vi "experiment description to file name Samuel.vi"(11 "Experiment Description":T1={"GAL4 Line / Line A / Genotype"="CS", "UAS-Effector Line / Line B"="", "Experiment Type"=enum."olfaction", "Stimulus Descriptions"=[{"Stimulus Modulation"=enum."Spatial", "stimulant"="co2", "maximum"=5, "mimimum"=0, "period"=20, "Modulation Detail"=enum."LinearX", "unit"="pct", "period_unit"="cm", "additional description"=enum."none", "description"=""}], "other name"="", "Training/Habituation Pre Exposure"={"CS"="", "UCS"="", "Training Protocol"="", "Training ID Code"="", "Training Type"=enum."none (no directory)"}}) -> (1 "data directory with time":path, 2 "filename":string, 3 "data directory":path)   [LabVIEW 2013]
panel:
  out "error out":errorcluster
  in  "error in":errorcluster
  # "X"
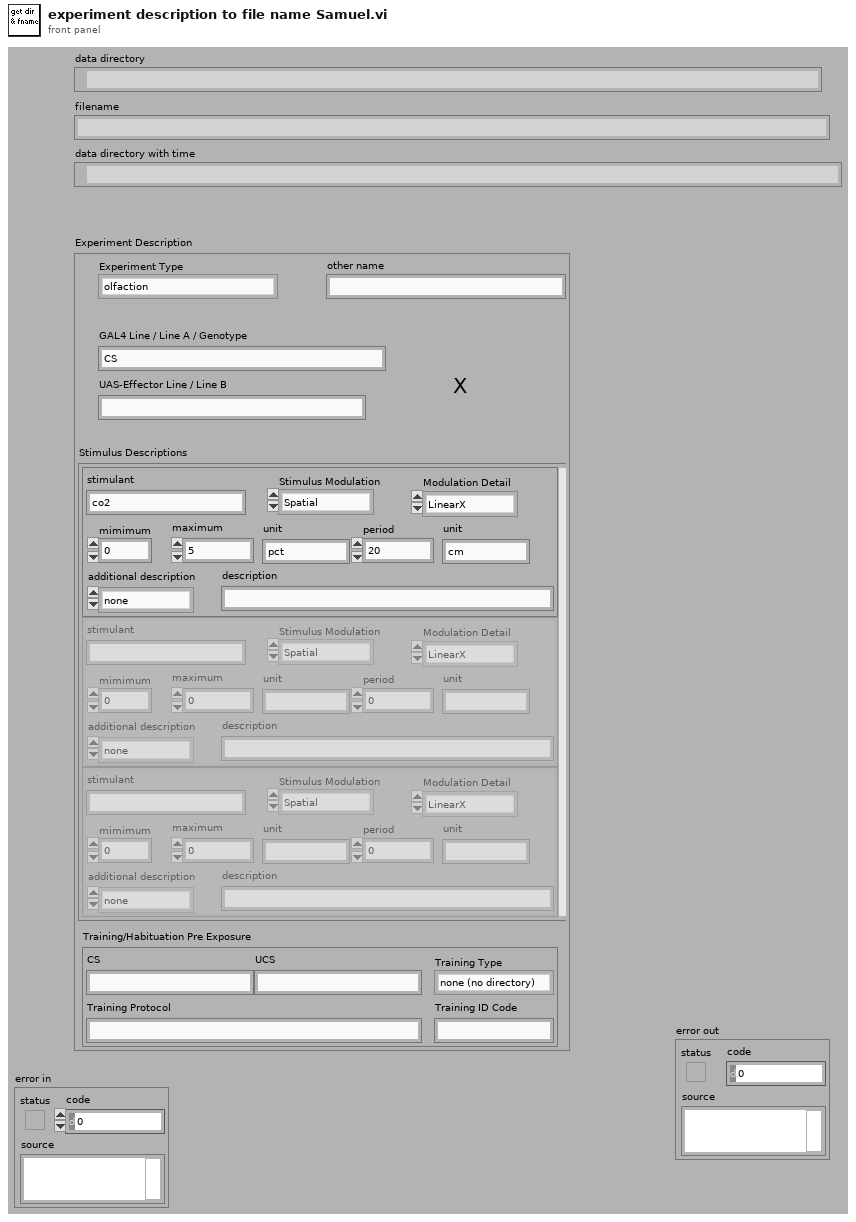
[diagram p1: front panel]
types:
  T1 = cluster{"GAL4 Line / Line A / Genotype":string, "UAS-Effector Line / Line B":string, "Experiment Type":enum16{"other", "olfaction", "phototaxis", "chemotaxis", "thermotaxis", "multi sensory"}, "Stimulus Descriptions":cluster{"Stimulus Modulation":enum16{"Spatial", "Temporal", "Constant", "Other"}, "stimulant":string, "maximum":u16, "mimimum":u16, "period":u16, "Modulation Detail":enum16{"LinearX", "LinearY", "Triangle", "Sine", "Square", "AngledX", "AngledY"}, "unit":string, "period_unit":string, "additional description":enum16{"none", "append", "replace"}, "description":string}[], "other name":string, "Training/Habituation Pre Exposure":cluster{"CS":string, "UCS":string, "Training Protocol":string, "Training ID Code":string, "Training Type":enum16{"none (no directory)", "untrained", "trained"}}}
  T2 = enum16{"other", "olfaction", "phototaxis", "chemotaxis", "thermotaxis", "multi sensory"}
  T3 = cluster{"Stimulus Modulation":enum16{"Spatial", "Temporal", "Constant", "Other"}, "stimulant":string, "maximum":u16, "mimimum":u16, "period":u16, "Modulation Detail":enum16{"LinearX", "LinearY", "Triangle", "Sine", "Square", "AngledX", "AngledY"}, "unit":string, "period_unit":string, "additional description":enum16{"none", "append", "replace"}, "description":string}[]
  T4 = cluster{"CS":string, "UCS":string, "Training Protocol":string, "Training ID Code":string, "Training Type":enum16{"none (no directory)", "untrained", "trained"}}
  T5 = enum16{"none (no directory)", "untrained", "trained"}
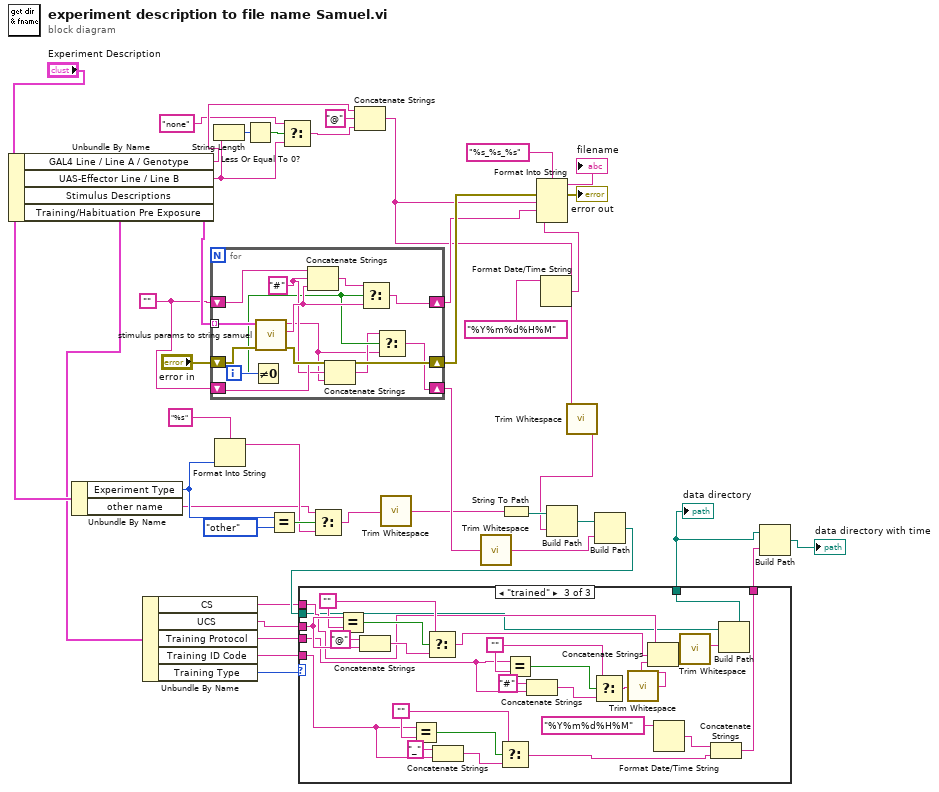
[diagram p0: block diagram]
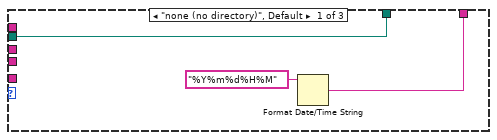
[diagram p2: hidden frame]
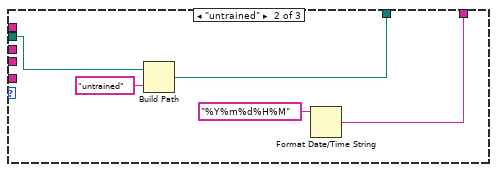
[diagram p3: hidden frame]
diagram:
  w20 = "" ("stimulus string description")
  n1 = Unbundle By Name("Experiment Description") -> ("GAL4 Line / Line A / Genotype"=w9:string, "UAS-Effector Line / Line B"=w4:string, "Stimulus Descriptions"=w41:T3, "Training/Habituation Pre Exposure"=w19:T4)
  n2 = Unbundle By Name("Experiment Description") -> ("Experiment Type"=w26:T2, "other name"=w21:string)
  n3 = Unbundle By Name(w19) -> ("CS"=w13:string, "UCS"=w12:string, "Training Protocol"=w11:string, "Training ID Code"=w10:string, "Training Type"=w18:T5)
  n4 = for {
    tunnel: w41 -> [w56] mode=indexing
    shift-right: [w54] -> w31
    shift-left: w20 -> [w53]
    shift-right: [w51] -> w39
    shift-left: "error in" -> [w50]
    shift-right: [w43] -> w6
    shift-left: w20 -> [w48]
    i -> [w55]
    w47 = "#"
    n5 = Not Equal To 0?(x=w55) -> (x != 0?=w46:bool)
    n6 = call "stimulus params to string samuel.vi"("error in"=w50, "stimulus params"=w56) -> ("error out"=w51:errorcluster, "short stimulus string"=w49:string, "stimulus string description"=w44:string)  [unwired: 7 in]
    n7 = Concatenate Strings(w53, w47, w49) -> (w52:string)
    n8 = Concatenate Strings(w48, w47, w44) -> (w45:string)
    n9 = Select(t=w52, s=w46, f=w49) -> (s? t:f=w54:string)
    n10 = Select(t=w45, s=w46, f=w44) -> (s? t:f=w43:string)
  }
  n11 = String Length(string=w4) -> (length=w29:i32)
  n12 = Format Into String(format string="%s", w26) -> (resulting string=w23:string)  [unwired: 2 in, 1 out]
  n13 = Less Or Equal To 0?(x=w29) -> (x <= 0?=w28:bool)
  n14 = Equal?(x=w26, y=T2."other") -> (x = y?=w24:bool)
  n15 = Select(t="none" ("f"), s=w28, f=w4) -> (s? t:f=w8:string)
  n16 = Select(t=w21, s=w24, f=w23) -> (s? t:f=w22:string)
  n17 = Concatenate Strings(w9, "@" ("string"), w8) -> (w7:string)
  n18 = call <vilib>:"Trim Whitespace.vi"("string"=w22) -> ("trimmed string"=w3:string)  [unwired: 1 in]
  n19 = call <vilib>:"Trim Whitespace.vi"("string"=w6) -> ("trimmed string"=w2:string)  [unwired: 1 in]
  n20 = String To Path(string=w3) -> (path=w34:path)
  n21 = Format Date/Time String(time format string (%c)="%Y%m%d%H%M") -> (date/time string=w30:string)  [unwired: 2 in]
  n22 = Format Into String(format string="%s_%s_%s", error in=w39, w7, w31, w30) -> (resulting string=→"filename":string, error out=→"error out":errorcluster)  [unwired: 1 in]
  n23 = call <vilib>:"Trim Whitespace.vi"("string"=w7) -> ("trimmed string"=w1:string)  [unwired: 1 in]
  n24 = Build Path(base path=w34, name or relative path=w1) -> (appended path=w33:path)
  n25 = Build Path(base path=w33, name or relative path=w2) -> (appended path=w17:path)
  n26 = case shown="\"trained\"" w18 {
    tunnel: w17 -> [w59 w64 w72]
    tunnel: [w59 w62 w71] -> w16
    tunnel: [w57 w60 w67] -> w15
    tunnel: w13 -> [_ _ w74]
    tunnel: w12 -> [_ _ w91]
    tunnel: w11 -> [_ _ w77]
    tunnel: w10 -> [_ _ w82]
    frame "none (no directory)", Default {
      n27 = Format Date/Time String(time format string (%c)="%Y%m%d%H%M") -> (date/time string=w57:string)  [unwired: 2 in]
    }
    frame "untrained" {
      n28 = Build Path(base path=w64, name or relative path="untrained") -> (appended path=w62:path)
      n29 = Format Date/Time String(time format string (%c)="%Y%m%d%H%M") -> (date/time string=w60:string)  [unwired: 2 in]
    }
    frame "trained" {
      w79 = ""
      w84 = ""
      w88 = ""
      n30 = Equal?(x=w91, y=w88) -> (x = y?=w89:bool)
      n31 = Concatenate Strings("@" ("string"), w91) -> (w87:string)
      n32 = Equal?(x=w82, y=w84) -> (x = y?=w85:bool)
      n33 = Select(t=w88, s=w89, f=w87) -> (s? t:f=w75:string)
      n34 = Concatenate Strings("_" ("string"), w82) -> (w83:string)
      n35 = Select(t=w84, s=w85, f=w83) -> (s? t:f=w68:string)
      n36 = Equal?(x=w77, y=w79) -> (x = y?=w80:bool)
      n37 = Concatenate Strings("#" ("string"), w77) -> (w78:string)
      n38 = Select(t=w79, s=w80, f=w78) -> (s? t:f=w76:string)
      n39 = call <vilib>:"Trim Whitespace.vi"("string"=w76) -> ("trimmed string"=w66:string)  [unwired: 1 in]
      n40 = Concatenate Strings(w74, w75, w66) -> (w73:string)
      n41 = Format Date/Time String(time format string (%c)="%Y%m%d%H%M") -> (date/time string=w69:string)  [unwired: 2 in]
      n42 = call <vilib>:"Trim Whitespace.vi"("string"=w73) -> ("trimmed string"=w65:string)  [unwired: 1 in]
      n43 = Concatenate Strings(w69, w68) -> (w67:string)
      n44 = Build Path(base path=w72, name or relative path=w65) -> (appended path=w71:path)
    }
  }
  "data directory" <- w16
  n45 = Build Path(base path=w16, name or relative path=w15) -> (appended path=→"data directory with time":path)
